vi "api_token_path.get.vi"(8 "error in (no error)":errorcluster, 11 "Nominal IO Client in":T1 format="%.0x") -> (0 "error out":errorcluster, 2 "API Token file":path, 3 "Nominal IO Client out":T1 format="%.0x", 4 "Found":bool)   [LabVIEW 2024, in "Nominal Client Scripting.lvlib"]
uses:
  Nominal Client Scripting.lvlib
  <vilib>/NI VeriStand/Custom Device API/Custom Device Item Ref.ctl
  <vilib>/NI VeriStand/Custom Device API/Get Item Property (Path).vi
  <vilib>/NI VeriStand/Custom Device API/Custom Device API.lvlib
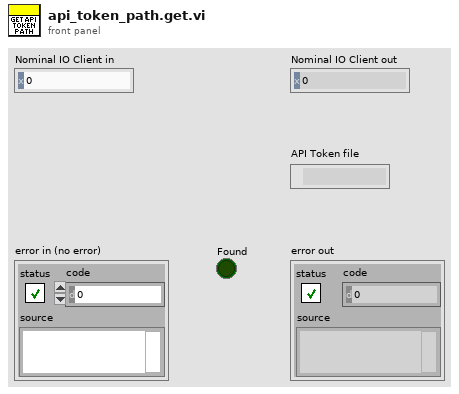
[diagram p1: front panel]
types:
  T1 = typedef "Custom Device API.lvlib/Custom Device Item Ref.ctl" = u64
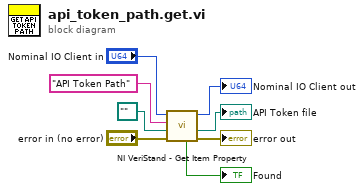
[diagram p0: block diagram]
diagram:
  n1 = call-poly <vilib>:"NI VeriStand - Get Item Property.vi"("error in (no error)"="error in (no error)", "Default Value"=path "", "Property Name"="API Token Path", "Item Ref in"="Nominal IO Client in") -> ("error out"=→"error out":errorcluster, "Value"=→"API Token file":path, "Item Ref out"=→"Nominal IO Client out":T1, "Found?"=→"Found":bool)  [unwired: 4 in]
